vi "GEA2 Initialize.vi"(0 "Board Index":i32, 5 "Source Address":u8=228 format="%.0x", 11 "error in":errorcluster) -> (4 "GEA Bus":refnum<k24>, 8 "Board ID":string, 15 "error out":errorcluster)   [LabVIEW 2014, in "GEA2_Toolkit.lvlib"]
doc: "This VI uses .NET DLLs to initialize a GEA2 connection over USB. The output is a reference to the newly opened GEA2 connection."
uses:
  library/GEA2_Toolkit.lvlib
  C:/Automation/DLLs/PC Tools .NET/GeaCommunication.dll
  Automation/DLLs/PC Tools .NET/GeaCommunication.dll
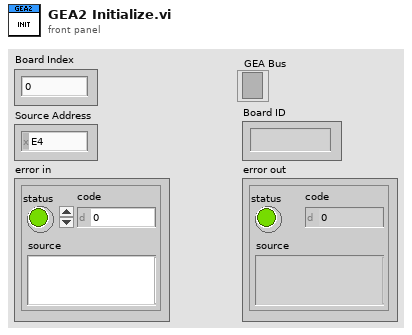
[diagram p1: front panel]
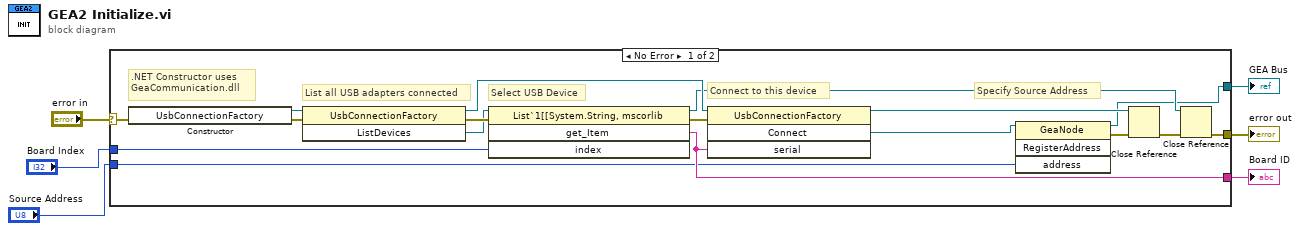
[diagram p0: block diagram]
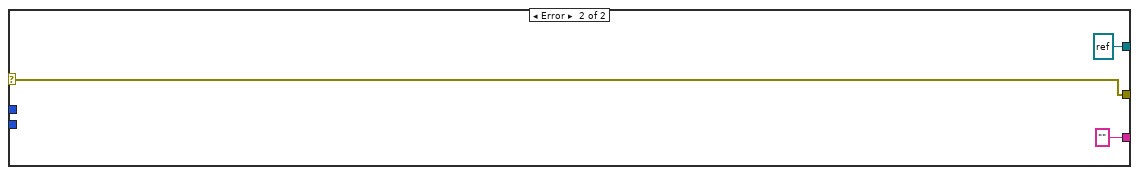
[diagram p2: hidden frame]
diagram:
  n1 = case shown="No Error" "error in" {
    selector: "error in" -> [w17 w26]
    tunnel: "Board Index" -> [w20 _]
    tunnel: [w11 w26] -> w6
    tunnel: [w7 refnum<k24> refnum ("Connect")] -> w1
    tunnel: "Source Address" -> [w9 _]
    tunnel: [w18 "" ("get_Item")] -> w2
    frame No Error {
      # "Specify Source Address"
      # "Connect to this device"
      # "Select USB Device"
      # "List all USB adapters connected"
      # ".NET Constructor uses\nGeaCommunication.dll"
      n2 = constructor class="UsbConnectionFactory"(error in=w17) -> (reference out=w14:refnum<k24>, error out=w16:errorcluster)  [unwired: 2 in, 1 out]
      n3 = invoke class="UsbConnectionFactory" method="ListDevices"(reference=w14, error in=w16) -> (reference out=w15:refnum<k24>, error out=w22:errorcluster, "ListDevices"=w21:refnum<k24>)  [unwired: 1 in]
      n4 = invoke class="List`1[[System.String, mscorlib" method="get_Item"(reference=w21, error in=w22, "index"=w20) -> (reference out=w13:refnum<k24>, error out=w23:errorcluster, "get_Item"=w18:string)  [unwired: 1 in, 1 out]
      n5 = invoke class="UsbConnectionFactory" method="Connect"(reference=w15, error in=w23, "serial"=w18) -> (reference out=w19:refnum<k24>, "Connect"=w10:refnum<k24>)  [unwired: 1 in, 2 out]
      n6 = invoke class="GeaNode" method="RegisterAddress"(reference=w10, "address"=w9) -> (reference out=w7:refnum<k24>, error out=w8:errorcluster)  [unwired: 2 in, 2 out]
      n7 = Close Reference(reference=w19, error in (no error)=w8) -> (error out=w12:errorcluster)
      n8 = Close Reference(reference=w13, error in (no error)=w12) -> (error out=w11:errorcluster)
    }
    frame Error {
    }
  }
  "error out" <- w6
  "Board ID" <- w2
  "GEA Bus" <- w1
